vi "Configuration Program.vi"(0 "VISA resource name":refnum<visa-resource-name>, 1 "Program Number (1)":i8=1 min=1 max=10 step=1, 2 "Short Channel (0:None)":u8(ring) items=["None", "Channel 1", "Channel 2", "Channel 3", "Channel 4", "Channel 5", "Channel 6", "Channel 7", "Channel 8 "], 3 "Active Channel (CH1-8 F:0)":T1, 4 "Chain (0)":i8 min=0 max=10, 5 "error in (no error)":errorcluster, 6 "ONTime (0.5 S)":sgl=0.5 min=0 format="%.4f", 7 "Sequence (1)":u8=1 min=1 max=10, 8 "Short Time (0.0 S)":sgl min=0 max=30 format="%.2f", 10 "OFFTime (0.0 S)":sgl min=0 format="%.4f", 11 "Sequence Mode (0:Skip)":u8(slide) scale=0.0..2.0, 12 "Run (F: Off)":bool, 13 "Save (T:Save)":bool=TRUE) -> (14 "VISA resource name out":refnum<visa-resource-name>, 19 "error out":errorcluster)   [LabVIEW 2015, in "Chroma ATE 6310.lvlib"]
doc: "Set the setting of the program.\n\nThe load is able to select customized basic tests,and link them into a program test for automatic execution.There are ten programs.Each programs has ten sequences to map files from 1 to 100."
uses:
  <instrlib>/Chroma ATE 6310/Chroma ATE 6310.lvlib
panel:
  # "Channel :       1          2          3          4           5          6          7          8"
  # "On\nOff"
  # "Save\nDon't Save"
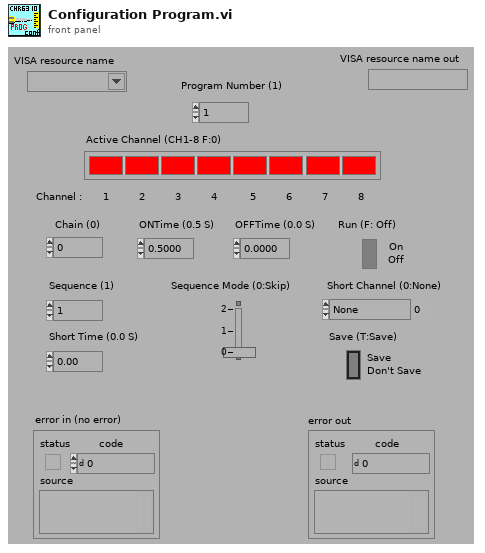
[diagram p1: front panel]
types:
  T1 = cluster{"CH1 (F:0)":bool, "CH2 (F:0)":bool, "CH3 (F:0)":bool, "CH4 (F:0)":bool, "CH5 (F:0)":bool, "CH6 (F:0)":bool, "CH7 (F:0)":bool, "CH8 (F:0)":bool}
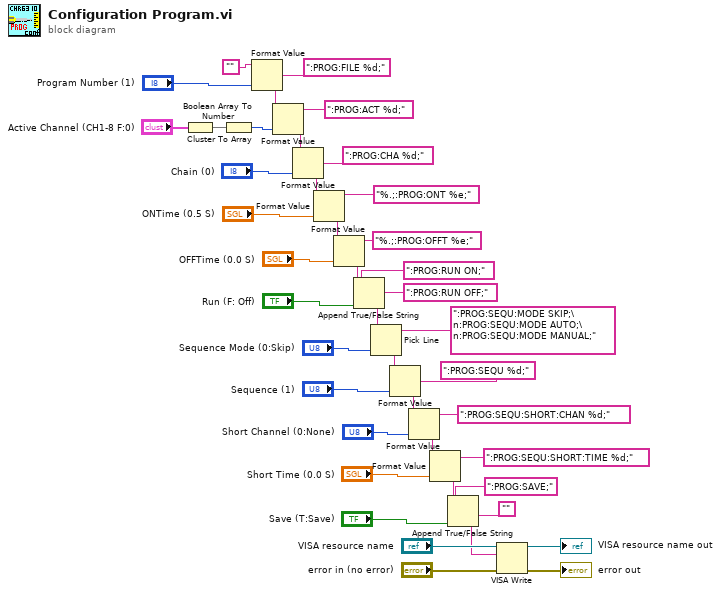
[diagram p0: block diagram]
diagram:
  n1 = Cluster To Array(cluster="Active Channel (CH1-8 F:0)") -> (array=w32:bool[])
  n2 = Boolean Array To Number(Boolean array=w32) -> (number=w30:u32)
  n3 = Format Value(string ("")="", format string=":PROG:FILE %d;", value (0)="Program Number (1)") -> (output string=w35:string)
  n4 = Format Value(string ("")=w35, format string=":PROG:ACT %d;", value (0)=w30) -> (output string=w19:string)
  n5 = Format Value(string ("")=w19, format string=":PROG:CHA %d;", value (0)="Chain (0)") -> (output string=w17:string)
  n6 = Format Value(string ("")=w17, format string="%.;:PROG:ONT %e;", value (0)="ONTime (0.5 S)") -> (output string=w24:string)
  n7 = Format Value(string ("")=w24, format string="%.;:PROG:OFFT %e;", value (0)="OFFTime (0.0 S)") -> (output string=w16:string)
  n8 = Append True/False String(1:"Run (F: Off)", 2:":PROG:RUN OFF;", 3:":PROG:RUN ON;", 4:w16) -> (0:w12:string)
  n9 = Pick Line(string ("")=w12, multi-line string=":PROG:SEQU:MODE SKIP;\n:PROG:SEQU:MODE AUTO;\n:PROG:SEQU:MODE MANUAL;", line index="Sequence Mode (0:Skip)") -> (output string=w10:string)
  n10 = Format Value(string ("")=w10, format string=":PROG:SEQU %d;", value (0)="Sequence (1)") -> (output string=w9:string)
  n11 = Format Value(string ("")=w9, format string=":PROG:SEQU:SHORT:CHAN %d;", value (0)="Short Channel (0:None)") -> (output string=w7:string)
  n12 = Format Value(string ("")=w7, format string=":PROG:SEQU:SHORT:TIME %d;", value (0)="Short Time (0.0 S)") -> (output string=w5:string)
  n13 = Append True/False String(1:"Save (T:Save)", 2:"", 3:":PROG:SAVE;", 4:w5) -> (0:w1:string)
  n14 = VISA Write(VISA resource name="VISA resource name", write buffer=w1, error in (no error)="error in (no error)") -> (VISA resource name out=→"VISA resource name out":refnum<visa-resource-name>, error out=→"error out":errorcluster)  [unwired: 1 out]
